vi "Update Command Data.vi"(8 "error in (no error)":errorcluster, 11 "Async Message in":refnum<class "Async Message.lvclass">) -> (0 "error out":errorcluster, 3 "Async Message out":refnum<class "Async Message.lvclass">)   [LabVIEW 2020, in "BCI-1553 API.lvlib" / "Async Message.lvclass"]
doc: "Updates the command data that will be written down to the Board. This method completely ignores all prior data stored in the Command Data parameter and updates it with the derived and masked data stored in this asynchrnous Message."
uses:
  Async Message.lvclass
  Async Message.lvclass/Async Message.ctl
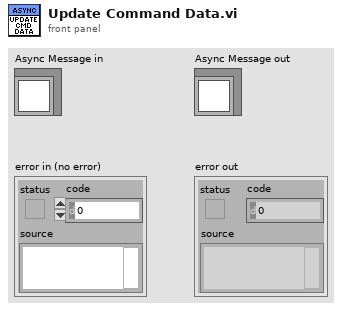
[diagram p1: front panel]
types:
  T1 = typedef "BCI-1553 API.lvlib/Command Type.ctl" = enum16{"Transmit", "Receive"}
  T2 = typedef "BCI-1553 API.lvlib/Command Word Count.ctl" = enum16{"1", "2", "3", "4", "5", "6", "7", "8", "9", "10", "11", "12", "13", "14", "15", "16", "17", "18", "19", "20", "21", "22", "23", "24", "25", "26", "27", "28", "29", "30", "31", "32"}
  T3 = typedef "BCI-1553 API.lvlib/Parameter Table Data.ctl" = cluster{"Parameter Name":string, "Base Word":u16, "Address":u16, "Value":u64, "Mask":u16[], "Scaling Info":T4}
  T4 = typedef "BCI-1553 API.lvlib/Scaling Information.ctl" = cluster{"Bit Offset":i32, "Bit Count":i32, "LSB Resolution":dbl, "2's Complement":bool, "Big Endian":bool, "Sign Bit":bool}
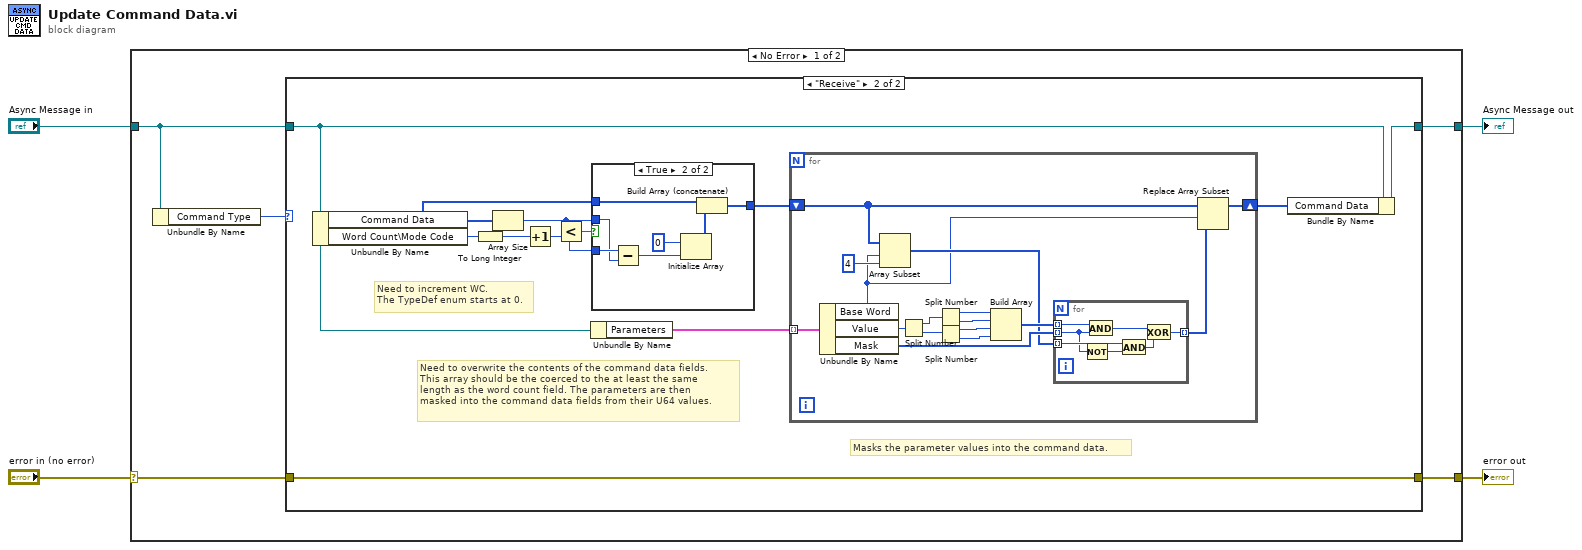
[diagram p0: block diagram]
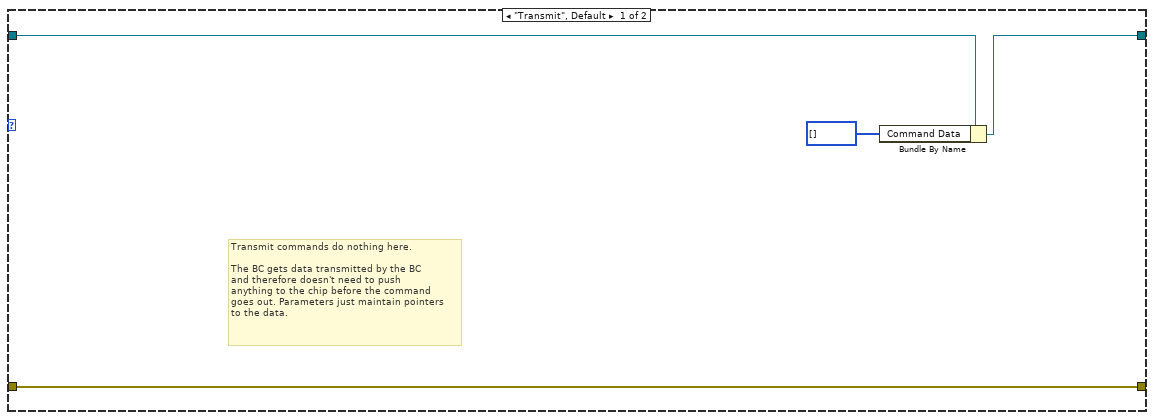
[diagram p2: hidden frame]
diagram:
  n1 = case shown="No Error" "error in (no error)" {
    selector: "error in (no error)" -> [w5 w58]
    tunnel: [w6 w58] -> w3
    tunnel: [w8 w57] -> w1
    tunnel: "Async Message in" -> [w7 w57]
    frame No Error {
      n2 = Unbundle By Name(w7) -> ("Command Type"=w9:T1)
      n3 = case shown="\"Receive\"" w9 {
        tunnel: [w11 w19] -> w8
        tunnel: w7 -> [w12 w18]
        tunnel: [w13 w25] -> w6
        tunnel: w5 -> [w13 w25]
        frame "Transmit", Default {
          # "Transmit commands do nothing here.\n\nThe BC gets data transmitted by the BC\nand therefore doesn't need to push\nanything to the chip before the command\ngoes out. Parameters just maintain pointers\nto the data."
          n4 = Bundle By Name(cluster=w12, "Command Data"=u16[] [] ("Async Message Config.Command Config.Command Data")) -> (w11:refnum<class "Async Message.lvclass">)
        }
        frame "Receive" {
          # "Need to increment WC.\nThe TypeDef enum starts at 0."
          # "Masks the parameter values into the command data."
          # "Need to overwrite the contents of the command data fields.\nThis array should be the coerced to the at least the same\nlength as the word count field. The parameters are then\nmasked into the command data fields from their U64 values."
          n5 = Unbundle By Name(w18) -> ("Command Data"=w22:u16[], "Word Count\\Mode Code"=w24:T2)
          n6 = To Long Integer(number=w24) -> (32bit integer=w21:i32)
          n7 = Array Size(array=w22) -> (size(s)=w20:i32)
          n8 = Increment(x=w21) -> (x+1=w14:i32)
          n9 = Less?(x=w20, y=w14) -> (x < y?=w23:bool)
          n10 = Unbundle By Name(w18) -> ("Parameters"=w15:T3[])
          n11 = case shown="True" w23 {
            tunnel: w22 -> [w49 w52]
            tunnel: w14 -> [_ w56]
            tunnel: w20 -> [_ w55]
            tunnel: [w49 w50] -> w17
            frame False {
            }
            frame True {
              n12 = Subtract(x=w56, y=w55) -> (x-y=w54:i32)
              n13 = Initialize Array(u16 0 ("Data"), w54) -> (w51:u16[])
              n14 = Build Array (concatenate)(w52, w51) -> (w50:u16[])
            }
          }
          n15 = for {
            shift-right: [w39] -> w16
            shift-left: w17 -> [w40]
            tunnel: w15 -> [w41] mode=indexing
            n16 = Unbundle By Name(w41) -> ("Base Word"=w26:u16, "Value"=w32:u64, "Mask"=w29:u16[])
            n17 = Array Subset(array=w40, index=w26, length=4) -> (w28:u16[])
            n18 = Split Number(x=w32) -> (hi(x)=w34:u32, lo(x)=w33:u32)
            n19 = Split Number(x=w34) -> (hi(x)=w35:u16, lo(x)=w36:u16)
            n20 = Split Number(x=w33) -> (hi(x)=w37:u16, lo(x)=w38:u16)
            n21 = Build Array(w35, w36, w37, w38) -> (w30:u16[])
            n22 = for {
              tunnel: w28 -> [w45] mode=indexing
              tunnel: w29 -> [w44] mode=indexing
              tunnel: w30 -> [w43] mode=indexing
              tunnel: [w42] -> w27 mode=indexing
              n23 = Not(x=w44) -> (.not. x?=w47:u16)
              n24 = And(x=w43, y=w44) -> (x .and. y?=w46:u16)
              n25 = And(x=w45, y=w47) -> (x .and. y?=w48:u16)
              n26 = Exclusive Or(1:w48, 2:w46) -> (0:w42:u16)
            }
            n27 = Replace Array Subset(array=w40, new element=w27, index=w26) -> (w39:u16[])
          }
          n28 = Bundle By Name(cluster=w18, "Command Data"=w16) -> (w19:refnum<class "Async Message.lvclass">)
        }
      }
    }
    frame Error {
    }
  }
  "error out" <- w3
  "Async Message out" <- w1
